vi "graph_cursor_1Darray.vi"(10 "Cusor list":T1, 11 "array in":dbl[](array[numeric])) -> (3 "array out":dbl[](array[numeric]))   [LabVIEW 2019]
uses:
  <vilib>/Utility/miscctls.llb/LVCursorListTypeDef.ctl
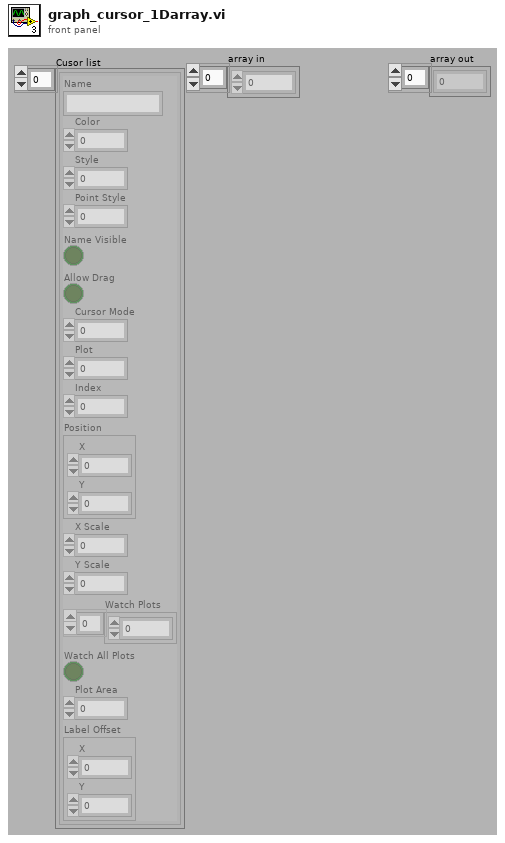
[diagram p1: front panel]
types:
  T1 = typedef "LVCursorListTypeDef.ctl" = cluster{"Name":string, "Color":u32, "Style":u8, "Point Style":u8, "Name Visible":bool, "Allow Drag":bool, "Cursor Mode":u32, "Plot":i32, "Index":i32, "Position":cluster{"X":dbl, "Y":dbl}, "X Scale":u32, "Y Scale":u32, "Watch Plots":i32[], "Watch All Plots":bool, "Plot Area":i32, "Label Offset":cluster{"X":dbl, "Y":dbl}}[]
  T2 = cluster{"Name":string, "Color":u32, "Style":u8, "Point Style":u8, "Name Visible":bool, "Allow Drag":bool, "Cursor Mode":u32, "Plot":i32, "Index":i32, "Position":cluster{"X":dbl, "Y":dbl}, "X Scale":u32, "Y Scale":u32, "Watch Plots":i32[], "Watch All Plots":bool, "Plot Area":i32, "Label Offset":cluster{"X":dbl, "Y":dbl}}
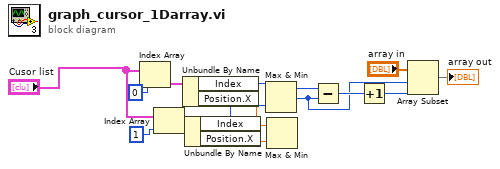
[diagram p0: block diagram]
diagram:
  n1 = Index Array(array="Cusor list", index=0) -> (element=w11:T2)
  n2 = Index Array(array="Cusor list", index=1) -> (element=w12:T2)
  n3 = Unbundle By Name(w11) -> ("Index"=w13:i32, "Position.X"=w6:dbl)
  n4 = Unbundle By Name(w12) -> ("Index"=w14:i32, "Position.X"=w5:dbl)
  n5 = Max & Min(x=w13, y=w14) -> (max(x,y)=w15:i32, min(x,y)=w7:i32)
  n6 = Max & Min(x=w6, y=w5) -> ()  [unwired: 2 out]
  n7 = Subtract(x=w15, y=w7) -> (x-y=w8:i32)
  n8 = Increment(x=w8) -> (x+1=w4:i32)
  n9 = Array Subset(array="array in", index=w7, length=w4) -> (→"array out":dbl[])
